vi "cource output offset.vi"(8 "error in (no error)":errorcluster, 11 "BME_DG_G08_Chnl in":refnum<class "BME_DG_G08_Chnl.lvclass">) -> (0 "error out":errorcluster, 1 "Output Offset":u32, 2 "OutputModulo":i32, 3 "BME_DG_G08_Chnl out":refnum<class "BME_DG_G08_Chnl.lvclass">)   [LabVIEW 2009, in "POLARIS BME DG.lvlib" / "BME_DG_G08_Chnl.lvclass"]
doc: "If cource output offset bit is set, this vi makes output offset = output modulo - 1.\nOther wise channel fires one trigger to late.\n\nauthor: Alexander Kessler, Helmholtz-Institut-Jena \nmaintainer: Alexander Kessler: alexander.kessler@uni-jena.de\n\nLast Change:\nLicense Agreement for this software:\n\nCopyright (C)\nHelmholtz-Institut-Jena\nFröbelsteg 3\n07743 Jena\nGermany\n\nContact: alexander.kessler@uni-jena.de\n\nThis program is free software; you can redistribute it and/or modify it under the terms of the GNU General Public License as published by the Free Software Foundation; either version 2 of the license, or (at your option) any later version.\n\nThis program is distributed in the hope that it will be useful, but WITHOUT ANY WARRANTY; without even the implied warranty of MERCHANTABILITY or FITNESS FOR A PARTICULAR PURPOSE. See the GNU General License for more details (http://www.gnu.org)."
uses:
  BME_DG_G08_Chnl.lvclass
  BME_DG_G08_Chnl.lvclass/BME_DG_G08_Chnl.ctl
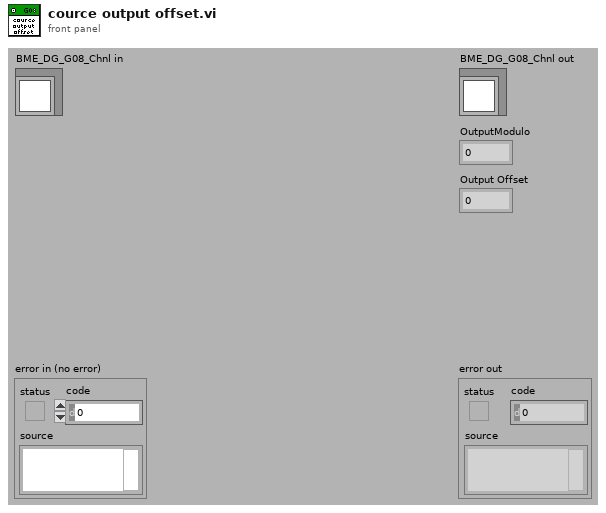
[diagram p1: front panel]
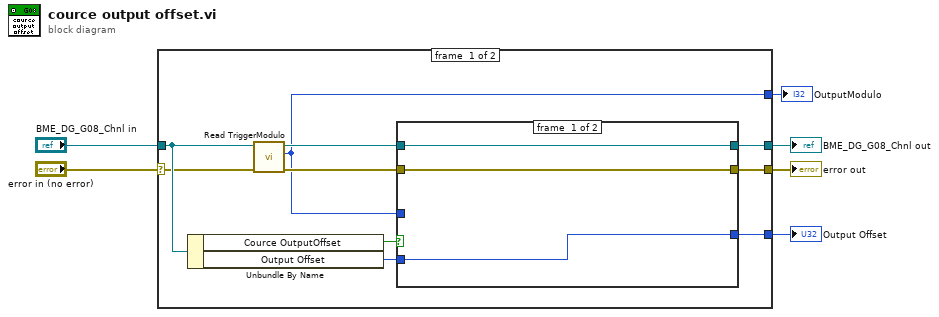
[diagram p0: block diagram]
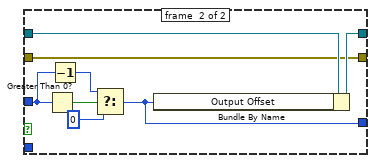
[diagram p2: hidden frame]
diagram:
  n1 = case shown="No Error" "error in (no error)" {
    selector: "error in (no error)" -> [w12 w29]
    tunnel: [w9 w29] -> w5
    tunnel: [w13 w28] -> w3
    tunnel: "BME_DG_G08_Chnl in" -> [w15 w28]
    tunnel: [w11 _] -> w2
    tunnel: [w7 _] -> w1
    frame #0 {
      n2 = Unbundle By Name(w15) -> ("Cource OutputOffset"=w16:bool, "Output Offset"=w10:u32)
      n3 = call-dynamic "Read TriggerModulo.vi"("error in (no error)"=w12, "BME_DG_G05_Chnl in"=w15) -> ("error out"=w8:errorcluster, "TriggerModulo"=w7:i32, "BME_DG_G05_Chnl out"=w14:refnum<class "BME_DG_G08_Chnl.lvclass">)  [unwired: 7 in]
      n4 = case shown="True" w16 {
        tunnel: w7 -> [_ w24]
        tunnel: w14 -> [w19 w27]
        tunnel: [w19 w26] -> w13
        tunnel: [w18 w21] -> w11
        tunnel: w10 -> [w18 _]
        tunnel: [w17 w20] -> w9
        tunnel: w8 -> [w17 w20]
        frame #0 {
        }
        frame #1 {
          n5 = Greater Than 0?(x=w24) -> (x > 0?=w25:bool)
          n6 = Decrement(x=w24) -> (x-1=w23:i32)
          n7 = Select(t=w23, s=w25, f=0) -> (s? t:f=w21:i32)
          n8 = Bundle By Name(cluster=w27, "Output Offset"=w21) -> (w26:refnum<class "BME_DG_G08_Chnl.lvclass">)
        }
      }
    }
    frame #1 {
    }
  }
  "error out" <- w5
  "BME_DG_G08_Chnl out" <- w3
  "Output Offset" <- w2
  "OutputModulo" <- w1
